vi "例6-11.vi"() -> ()   [LabVIEW 2019]
uses:
  <vilib>/Analysis/2dsp.llb/Real FFT.vi
  <vilib>/Analysis/NI_AALPro.lvlib
  <vilib>/Analysis/NI_AALBase.lvlib
panel:
  in  "采样点数":dbl=100.0
  in  "采样频率":dbl=100.0
  in  "幅值2":dbl=2.0
  in  "频率2":dbl=20.0
  in  "幅值1":dbl=1.0
  in  "频率1":dbl=10.0
  out "频域波形":cluster{i32, dbl, dbl[]}(graph)
  out "时域波形":cluster{i32, dbl, dbl[]}(graph)
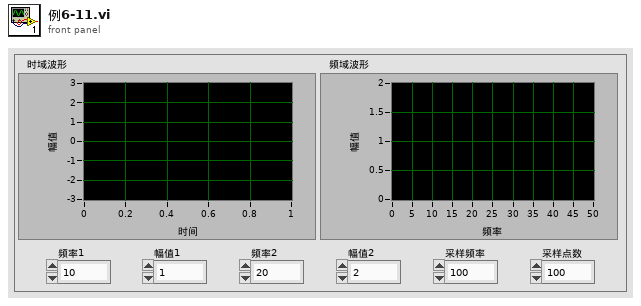
[diagram p1: front panel]
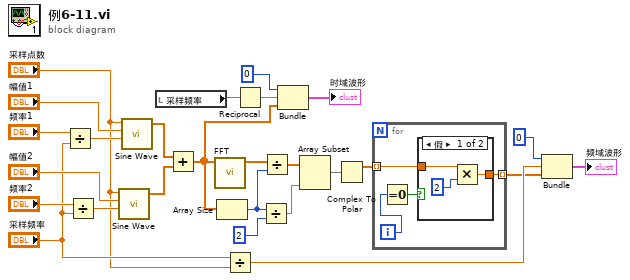
[diagram p0: block diagram]
diagram:
  n1 = Divide(x="频率1", y="采样频率") -> (x/y=w23:dbl)
  n2 = Divide(x="频率2", y="采样频率") -> (x/y=w24:dbl)
  n3 = call <vilib>:"Sine Wave.vi"("samples"="采样点数", "amplitude"="幅值2", "frequency"=w24) -> ("sine wave"=w19:dbl[])  [unwired: 2 in, 2 out]
  n4 = call <vilib>:"Sine Wave.vi"("samples"="采样点数", "amplitude"="幅值1", "frequency"=w23) -> ("sine wave"=w20:dbl[])  [unwired: 2 in, 2 out]
  n5 = local read "采样频率"() -> (w17:dbl)
  n6 = Add(x=w20, y=w19) -> (x+y=w14:dbl[])
  n7 = call-poly <vilib>:"FFT.vi"("X"=w14) -> ("FFT {X}"=w13:cdb[])  [unwired: 9 in, 1 out]
  n8 = Array Size(array=w14) -> (size(s)=w7:i32)
  n9 = Divide(x="采样频率", y="采样点数") -> (x/y=w11:dbl)
  n10 = Reciprocal(x=w17) -> (1/x=w16:dbl)
  n11 = Divide(x=w7, y=2) -> (x/y=w4:dbl)
  n12 = Divide(x=w13, y=w7) -> (x/y=w5:cdb[])
  n13 = Bundle(0, w16, w14) -> (→"时域波形":cluster{i32, dbl, dbl[]})  [unwired: 1 in]
  n14 = Array Subset(array=w5, length=w4) -> (w3:cdb[])  [unwired: 1 in]
  n15 = Complex To Polar(r * e^(i*theta)=w3) -> (r=w2:dbl[])  [unwired: 1 out]
  n16 = for {
    tunnel: w2 -> [w28] mode=indexing
    tunnel: [w27] -> w1 mode=indexing
    i -> [w29]
    n17 = Equal To 0?(x=w29) -> (x = 0?=w30:bool)
    n18 = case shown="假" w30 {
      tunnel: w28 -> [w32 w34]
      tunnel: [w31 w34] -> w27
      frame False {
        n19 = Multiply(x=w32, y=2) -> (x*y=w31:dbl)
      }
      frame True {
      }
    }
  }
  n20 = Bundle(0, w11, w1) -> (→"频域波形":cluster{i32, dbl, dbl[]})  [unwired: 1 in]
